vi "Get_IT_Hole.vi"(0 "Data Cluster":T1 {"Shaft"."dmin" format="%#_7g"; "Shaft"."dmax" format="%#_7g"; "Shaft"."Fundamental Dev" format="%#_7g"; "Shaft"."Tolerance Grade (IT) Shaft" format="%#_7g"; "Hole"."Dmin" format="%#_7g"; "Hole"."Tolerance Grade (IT)" format="%#_7g"}, 3 "error in (no error)":errorcluster) -> (5 "Data Cluster Out":T1 {"Shaft"."dmin" format="%#_7g"; "Shaft"."dmax" format="%#_7g"; "Shaft"."Fundamental Dev" format="%#_7g"; "Shaft"."Tolerance Grade (IT) Shaft" format="%#_7g"; "Hole"."Dmin" format="%#_7g"; "Hole"."Tolerance Grade (IT)" format="%#_7g"}, 7 "error out":errorcluster)   [LabVIEW 2023]
uses:
  TypeDef/Data_Cluster.ctl
  TypeDef/Units.ctl
  TypeDef/Method_Info.ctl
  TypeDef/Hole_Data.ctl
  TypeDef/Shaft_Data.ctl
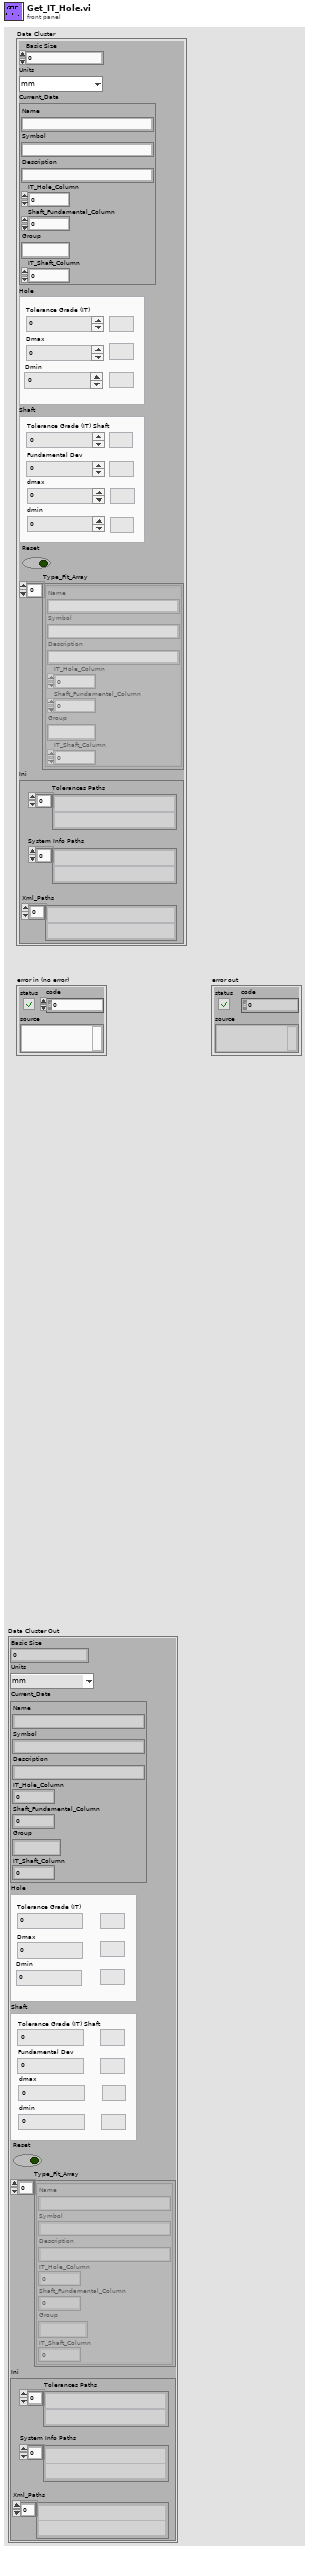
[diagram p1: front panel]
types:
  T1 = typedef "Data_Cluster.ctl" = cluster{"Basic Size ":dbl, "Units":T2, "Current_Data":T3, "Hole":T4, "Shaft":T5, "Reset":bool, "Type_Fit_Array":T3[], "Ini":cluster{"Tolerances Paths":path[], "System Info Paths":path[], "Xml_Paths":path[]}}
  T2 = typedef "Units.ctl" = enum16{"mm", "in"}
  T3 = typedef "Method_Info.ctl" = cluster{"Name":string, "Symbol":string, "Description":string, "IT_Hole_Column":i32, "Shaft_Fundamental_Column":i32, "Group":string, "IT_Shaft_Column":i32}
  T4 = typedef "Hole_Data.ctl" = cluster{"Tolerance Grade (IT)":dbl, "Dmax":dbl, "Units Hole":cluster{"units_it":string, "units_Dmax\nUnits_Dmax":string, "Units_Dmin":string}, "Dmin":dbl}
  T5 = typedef "Shaft_Data.ctl" = cluster{"Tolerance Grade (IT) Shaft":dbl, "Units Shaft":cluster{"Units_FundamentalDev":string, "Units_dmax":string, "Units_dmin":string, "Units_IT_Shaft":string}, "Fundamental Dev":dbl, "dmax":dbl, "dmin":dbl}
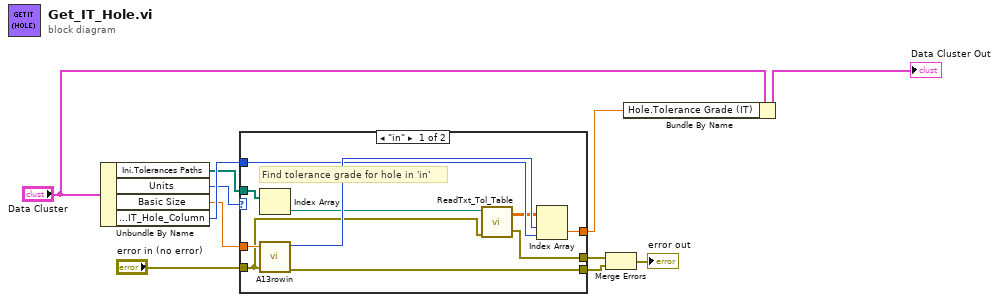
[diagram p0: block diagram]
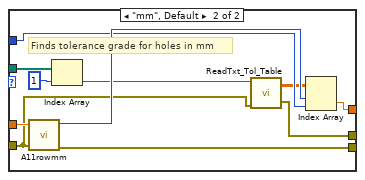
[diagram p2: hidden frame]
diagram:
  n1 = Unbundle By Name("Data Cluster") -> ("Ini.Tolerances Paths"=w7:path[], "Units"=w4:T2, "Basic Size"=w6:dbl, "Current_Data.IT_Hole_Column"=w8:i32)
  n2 = case shown="\"in\"" w4 {
    tunnel: "error in (no error)" -> [w14 w26]
    tunnel: [w16 w29] -> w1
    tunnel: w6 -> [w21 w32]
    tunnel: w7 -> [w20 w24]
    tunnel: w8 -> [w17 w30]
    tunnel: [w13 w25] -> w9
    tunnel: [w19 w28] -> w10
    frame "in" {
      # "Find tolerance grade for hole in 'in'"
      n3 = Index Array(array=w20) -> (element=w12:path)  [unwired: 1 in]
      n4 = call "A13rowin.vi"("Basic Size"=w21, "error in"=w14) -> ("Row"=w18:i32, "error out"=w19:errorcluster)  [unwired: 5 in]
      n5 = call "ReadTxt_Tol_Table.vi"("error in"=w14, "ITmm path"=w12) -> ("error out"=w13:errorcluster, "array_of_tolerances"=w15:dbl[][])  [unwired: 4 in]
      n6 = Index Array(array=w15, index (row)=w18, index (col)=w17) -> (element=w16:dbl)
    }
    frame "mm", Default {
      # "Finds tolerance grade for holes in mm"
      n7 = call "A11rowmm.vi"("Basic Size"=w32, "error in (no error)"=w26) -> ("Row"=w31:i32, "error out"=w28:errorcluster)  [unwired: 5 in]
      n8 = Index Array(array=w24, index=1) -> (element=w22:path)
      n9 = call "ReadTxt_Tol_Table.vi"("error in"=w26, "ITmm path"=w22) -> ("error out"=w25:errorcluster, "array_of_tolerances"=w27:dbl[][])  [unwired: 4 in]
      n10 = Index Array(array=w27, index (row)=w31, index (col)=w30) -> (element=w29:dbl)
    }
  }
  n11 = Merge Errors(w9, w10) -> (→"error out":errorcluster)
  n12 = Bundle By Name(cluster="Data Cluster", "Hole.Tolerance Grade (IT)"=w1) -> (→"Data Cluster Out":T1)
